vi "Contour2Pic.vi"(8 "Hdist":dbl, 9 "Vpix":u32, 10 "Hpix":u32, 11 "Polys":T1[](array[typedef])) -> (3 "Pic":picture)   [LabVIEW 2014]
uses:
  TypeDefs/Poly2DwSlope.ctl
  TypeDefs/Point2DwSlope.ctl
  TypeDefs/Line2D.ctl
  <vilib>/picture/picture.llb/Draw True-Color Pixmap.vi
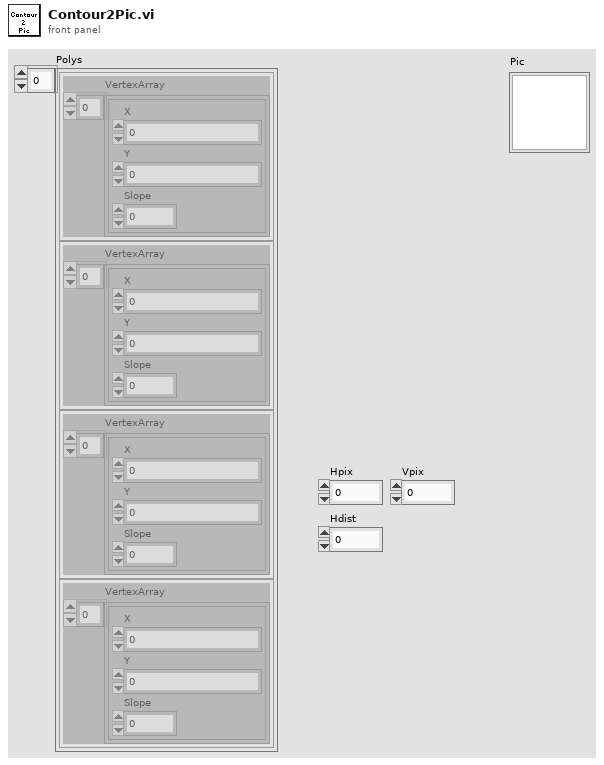
[diagram p1: front panel]
types:
  T1 = typedef "Poly2DwSlope.ctl" = cluster{"VertexArray":T2[]}
  T2 = typedef "Point2DwSlope.ctl" = cluster{"X":sgl, "Y":sgl, "Slope":dbl}
  T3 = typedef "Line2D.ctl" = cluster{"Vertex1":T2, "Vertex2":T2, "Slope":dbl}
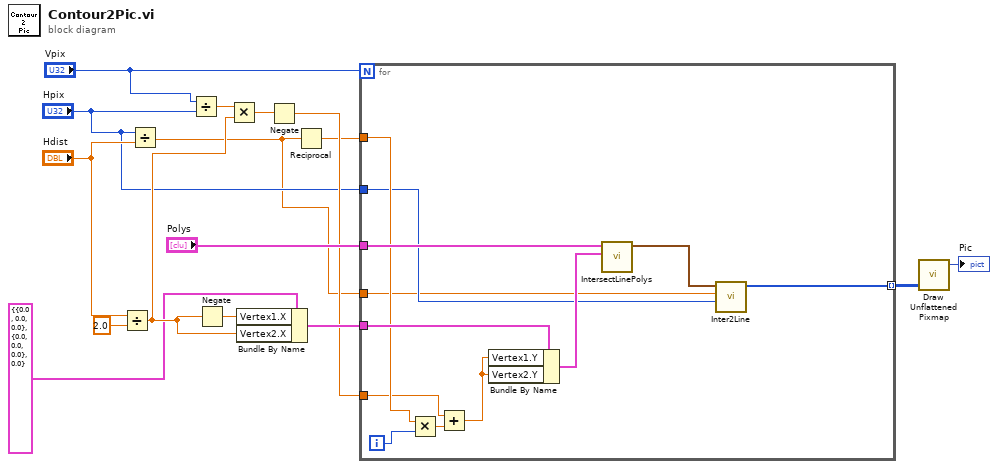
[diagram p0: block diagram]
diagram:
  n1 = Divide(x="Hdist", y=2.0) -> (x/y=w8:dbl)
  n2 = Divide(x="Hpix", y="Hdist") -> (x/y=w5:dbl)
  n3 = Divide(x="Vpix", y="Hpix") -> (x/y=w13:dbl)
  n4 = Negate(x=w8) -> (-x=w15:dbl)
  n5 = Multiply(x=w13, y=w8) -> (x*y=w12:dbl)
  n6 = Bundle By Name(cluster=T3 {"Vertex1"={"X"=0.0, "Y"=0.0, "Slope"=0.0}, "Vertex2"={"X"=0.0, "Y"=0.0, "Slope"=0.0}, "Slope"=0.0} ("Line2D"), "Vertex1.X"=w15, "Vertex2.X"=w8) -> (w14:T3)
  n7 = Negate(x=w12) -> (-x=w11:dbl)
  n8 = Reciprocal(x=w5) -> (1/x=w7:dbl)
  n9 = for {
    N: "Vpix" -> [_]
    tunnel: "Polys" -> [w28]
    tunnel: w14 -> [w27]
    tunnel: w7 -> [w26]
    tunnel: w11 -> [w23]
    tunnel: "Hpix" -> [w19]
    tunnel: w5 -> [w18]
    tunnel: [w17] -> w4 mode=indexing
    i -> [w25]
    n10 = Multiply(x=w26, y=w25) -> (x*y=w24:dbl)
    n11 = Add(x=w23, y=w24) -> (x+y=w22:dbl)
    n12 = Bundle By Name(cluster=w27, "Vertex1.Y"=w22, "Vertex2.Y"=w22) -> (w21:T3)
    n13 = call "IntersectLinePolys.vi"("Line2D"=w21, "Polys"=w28) -> ("Intersections"=w20:T2[])  [unwired: 9 in]
    n14 = call "Inter2Line.vi"("Length"=w19, "Scaling(dist/pix)"=w18, "Intersections"=w20) -> ("FilledLine"=w17:u32[])  [unwired: 8 in]
  }
  n15 = call-poly <vilib>:"Draw Unflattened Pixmap.vi"("data (RGB format)"=w4) -> ("new picture"=→"Pic":picture)  [unwired: 8 in]
